vi "Ejercicio 3.5.vi"() -> ()   [LabVIEW 2021]
panel:
  out "Waveform Graph":cluster{i32, dbl, dbl[]}(graph)
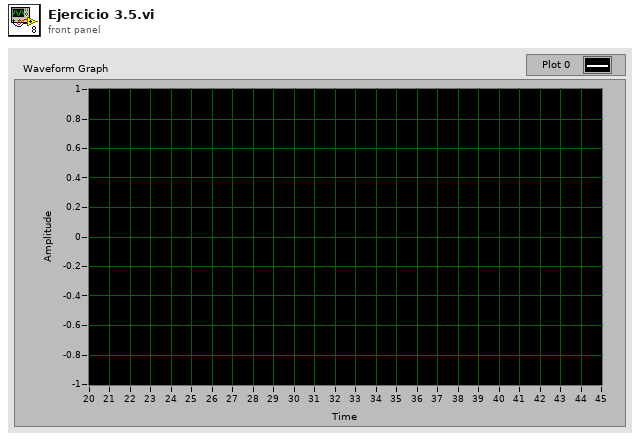
[diagram p1: front panel]
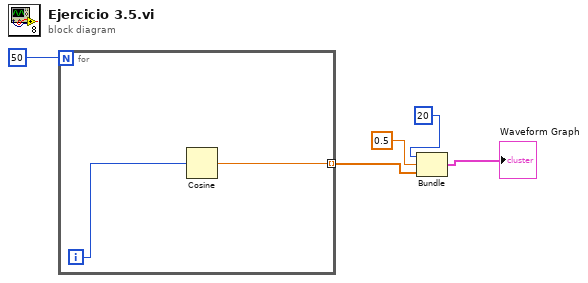
[diagram p0: block diagram]
diagram:
  n1 = for {
    N: 50 -> [_]
    tunnel: [w6] -> w4 mode=indexing
    i -> [w7]
    n2 = Cosine(x=w7) -> (cos(x)=w6:dbl)
  }
  n3 = Bundle(20, 0.5, w4) -> (→"Waveform Graph":cluster{i32, dbl, dbl[]})  [unwired: 1 in]
